vi "Initialize JSON Schema.vi"(8 "error in (no error)":errorcluster, 9 "Description":string, 10 "Title":string, 11 "JSON Schema in":string="{}") -> (0 "error out":errorcluster, 3 "JSON Schema out":string)   [LabVIEW 2019, in "JSON-Schema.lvlib"]
doc: "Initialize a JSON Schema with <b>Title</b> and <b>Description</b>\n\nSets JSON Schema Dialect to draft 2020-12."
uses:
  JSON-Schema.lvlib
  typedefs/JSON Schema Dialect--Enum.ctl
  da36fd2b-f3e2-4667-bfdb-8686c9034e16.vi
  773a2bdd-5bb6-4476-aa24-30e852a44520.vi
  <vilib>/JDP Science/JSONtext/Variant to JSON Text.vi
  <vilib>/JDP Science/JSONtext/Set Item.vi
  <vilib>/JDP Science/JSONtext/LVClass Serializer/JSONtext LVClass Serializer.lvclass
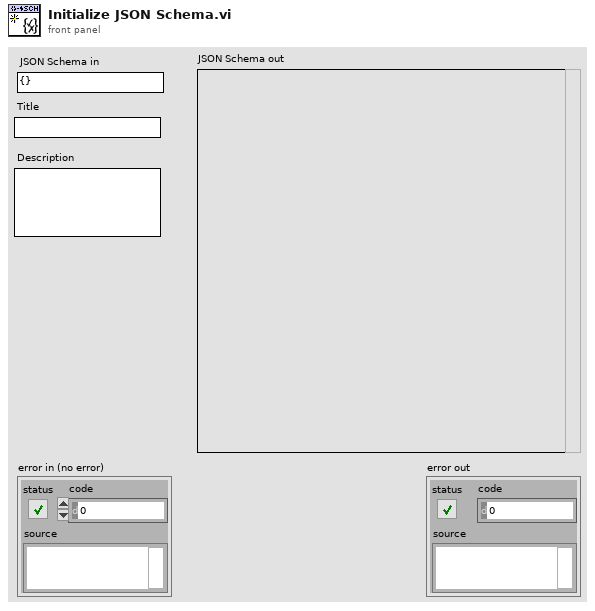
[diagram p1: front panel]
types:
  T1 = typedef "JSON-Schema.lvlib/JSON Schema Dialect--Enum.ctl" = enum16{"2020-12", "2019-09", "draft-07", "draft-06", "draft-05", "custom"}
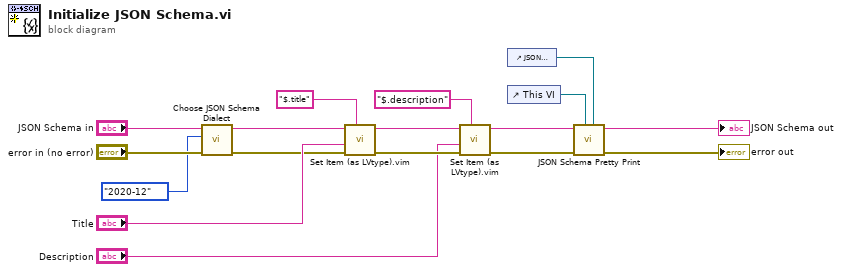
[diagram p0: block diagram]
diagram:
  n1 = call "Choose JSON Schema Dialect.vi"("error in (no error)"="error in (no error)", "Dialect"=JSON_Schema_Dialect--Enum."2020-12" ("JSON Schema Dialect"), "JSON Schema in"="JSON Schema in") -> ("error out"=w5:errorcluster, "JSON Schema out"=w4:string)  [unwired: 7 in]
  n2 = call "Set Item (as LVtype).vim"("$Path or Item Name"="$.title", "error in (no error)"=w5, "Anything"="Title", "JSON"=w4) -> ("error out"=w12:errorcluster, "<JSON>"=w13:string)  [unwired: 4 in, 1 out]
  n3 = call "Set Item (as LVtype).vim"("$Path or Item Name"="$.description", "error in (no error)"=w12, "Anything"="Description", "JSON"=w13) -> ("error out"=w9:errorcluster, "<JSON>"=w3:string)  [unwired: 4 in, 1 out]
  n4 = control-ref of="JSON Schema out"() -> (w1:refnum<vi>)
  n5 = control-ref of="This VI"() -> (w2:refnum<vi>)
  n6 = call "JSON Schema Pretty Print.vi"("String Control"=w1, "reference"=w2, "error in (no error)"=w9, "<JSON> in"=w3) -> ("error out"=→"error out":errorcluster, "<JSON> out"=→"JSON Schema out":string)  [unwired: 6 in]
